vi "简易流程路径写入.vi"(8 "error in (no error)":errorcluster caption="错误输入（无错误）", 10 "简易流程路径":path, 11 "Cleaningcycle 输入":refnum<class "Cleaning cycle.lvclass">) -> (0 "error out":errorcluster caption="错误输出", 3 "Cleaningcycle 输出":refnum<class "Cleaning cycle.lvclass">)   [LabVIEW 2016, in "Cleaning cycle.lvclass"]
uses:
  Cleaning cycle.lvclass
  Cleaning cycle.lvclass/Cleaning cycle.ctl
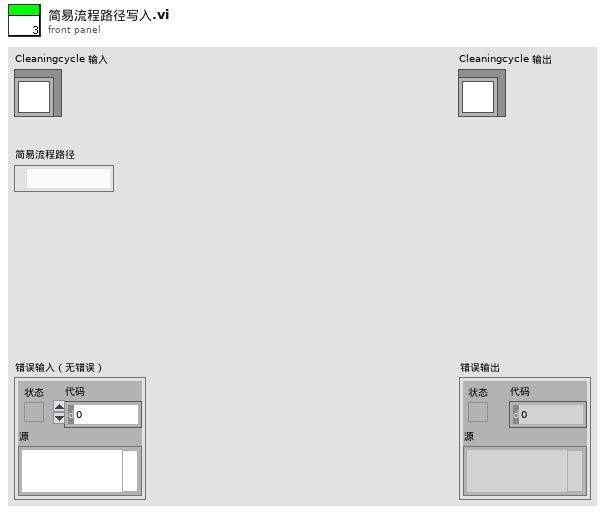
[diagram p1: front panel]
types:
  T1 = typedef "Cleaning cycle.lvclass/State Data.ctl" = cluster{"配置文件路径":path, "简易流程路径":path, "参数列表":cluster{"String":string, "Value":u16}[], "简易流程列表":cluster{"String":string, "Value":u16}[], "配置信息":T2, "命令":cluster{"触发":bool, "周期项":T4}[]}
  T2 = typedef "Cleaning cycle.lvclass/配置信息.ctl" = cluster{"任务列表":T3}
  T3 = typedef "Cleaning cycle.lvclass/任务.ctl" = cluster{"启用":bool, "项":string[][]}
  T4 = typedef "Cleaning cycle.lvclass/周期项.ctl" = cluster{"时":i32, "分":i32, "频次":string, "id":i32, "参数":string, "simpleflowid":i32, "简易流程名称":string}
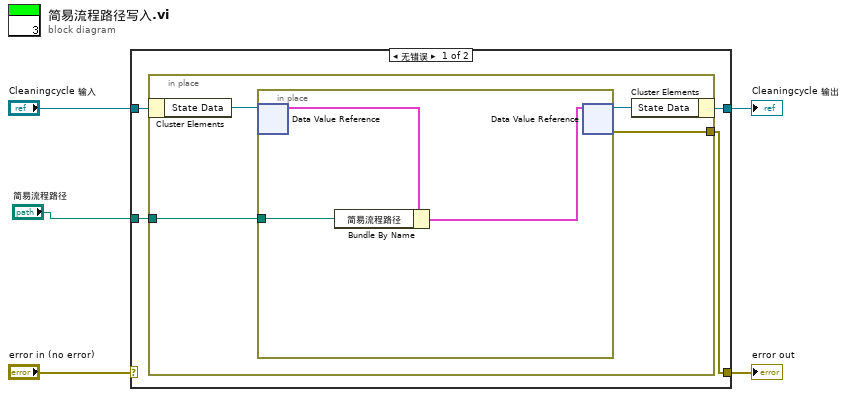
[diagram p0: block diagram]
diagram:
  n1 = case shown="无错误" "error in (no error)" {
    selector: "error in (no error)" -> [_ w18]
    tunnel: [w7 w18] -> w4
    tunnel: [w8 w17] -> w2
    tunnel: "Cleaningcycle 输入" -> [w9 w17]
    tunnel: "简易流程路径" -> [w6 _]
    frame No Error {
      n2 = in-place {
        in-place-border: [w11] -> w7
        in-place-border: w6 -> [w10]
        n3 = in-place-cluster #1(w9) -> ("State Data"=w13:refnum<data-value>)
        n4 = in-place {
          in-place-border: w10 -> [w14]
          n5 = in-place-dvr #2(w13) -> (w16:T1)  [unwired: 1 out]
          n6 = Bundle By Name(cluster=w16, "简易流程路径"=w14) -> (w15:T1)
          n7 = in-place-dvr #2(w15) -> (w12:refnum<data-value>, w11:errorcluster)
        }
        n8 = in-place-cluster #1("State Data"=w12) -> (w8:refnum<class "Cleaning cycle.lvclass">)
      }
    }
    frame Error {
    }
  }
  "error out" <- w4
  "Cleaningcycle 输出" <- w2
